vi "Database.Select.Variant.vi"(8 "error in":errorcluster, 9 "System":string="ST10", 10 "Variant":u64, 11 "Data in":T1 {"Variant"."TS"."TV"."minimum" format="%#.3f"; "Variant"."TS"."TV"."maximum" format="%#.3f"; "Variant"."TS"."TP"."value" format="%#.3f"}) -> (0 "error out":errorcluster, 3 "Data out":T1 {"Variant"."TS"."TV"."minimum" format="%#.3f"; "Variant"."TS"."TV"."maximum" format="%#.3f"; "Variant"."TS"."TP"."value" format="%#.3f"})   [LabVIEW 2016]
doc: "Write test results (measurement values) to proda database\n\nWabco 2017 All right reserved\nAuthor: maciej.szupienko@wabco-auto.com"
uses:
  Database.Main.Data.ctl
  Database.Main.Data.Status.ctl
  Database.Main.Data.Sets.ctl
  Database.Main.Data.Results.ctl
  ProdaNG/Controls/ProdaNG.Identification.ctl
  ProdaNG/Controls/ProdaNG.ProcessResult.ctl
  ProdaNG/Controls/ProdaNG.ProcessStepResult.ctl
  ProdaNG/Controls/ProdaNG.TestStepResult.ctl
  ProdaNG/Controls/ProdaNG.TestValueResult.ctl
  Database.Main.Data.Variant.ctl
  ProdaNG/Controls/ProdaNG.ProcessStepParam.ctl
  ProdaNG/Controls/ProdaNG.TestStep.ctl
  ProdaNG/Controls/ProdaNG.TestStepParam.ctl
  ProdaNG/Controls/ProdaNG.TestValue.ctl
  tools/Translator/Translator.Message.ctl
  tools/EventLog/EventLog.EventSource.ctl
  tools/EventLog/EventLog.New(single).vi
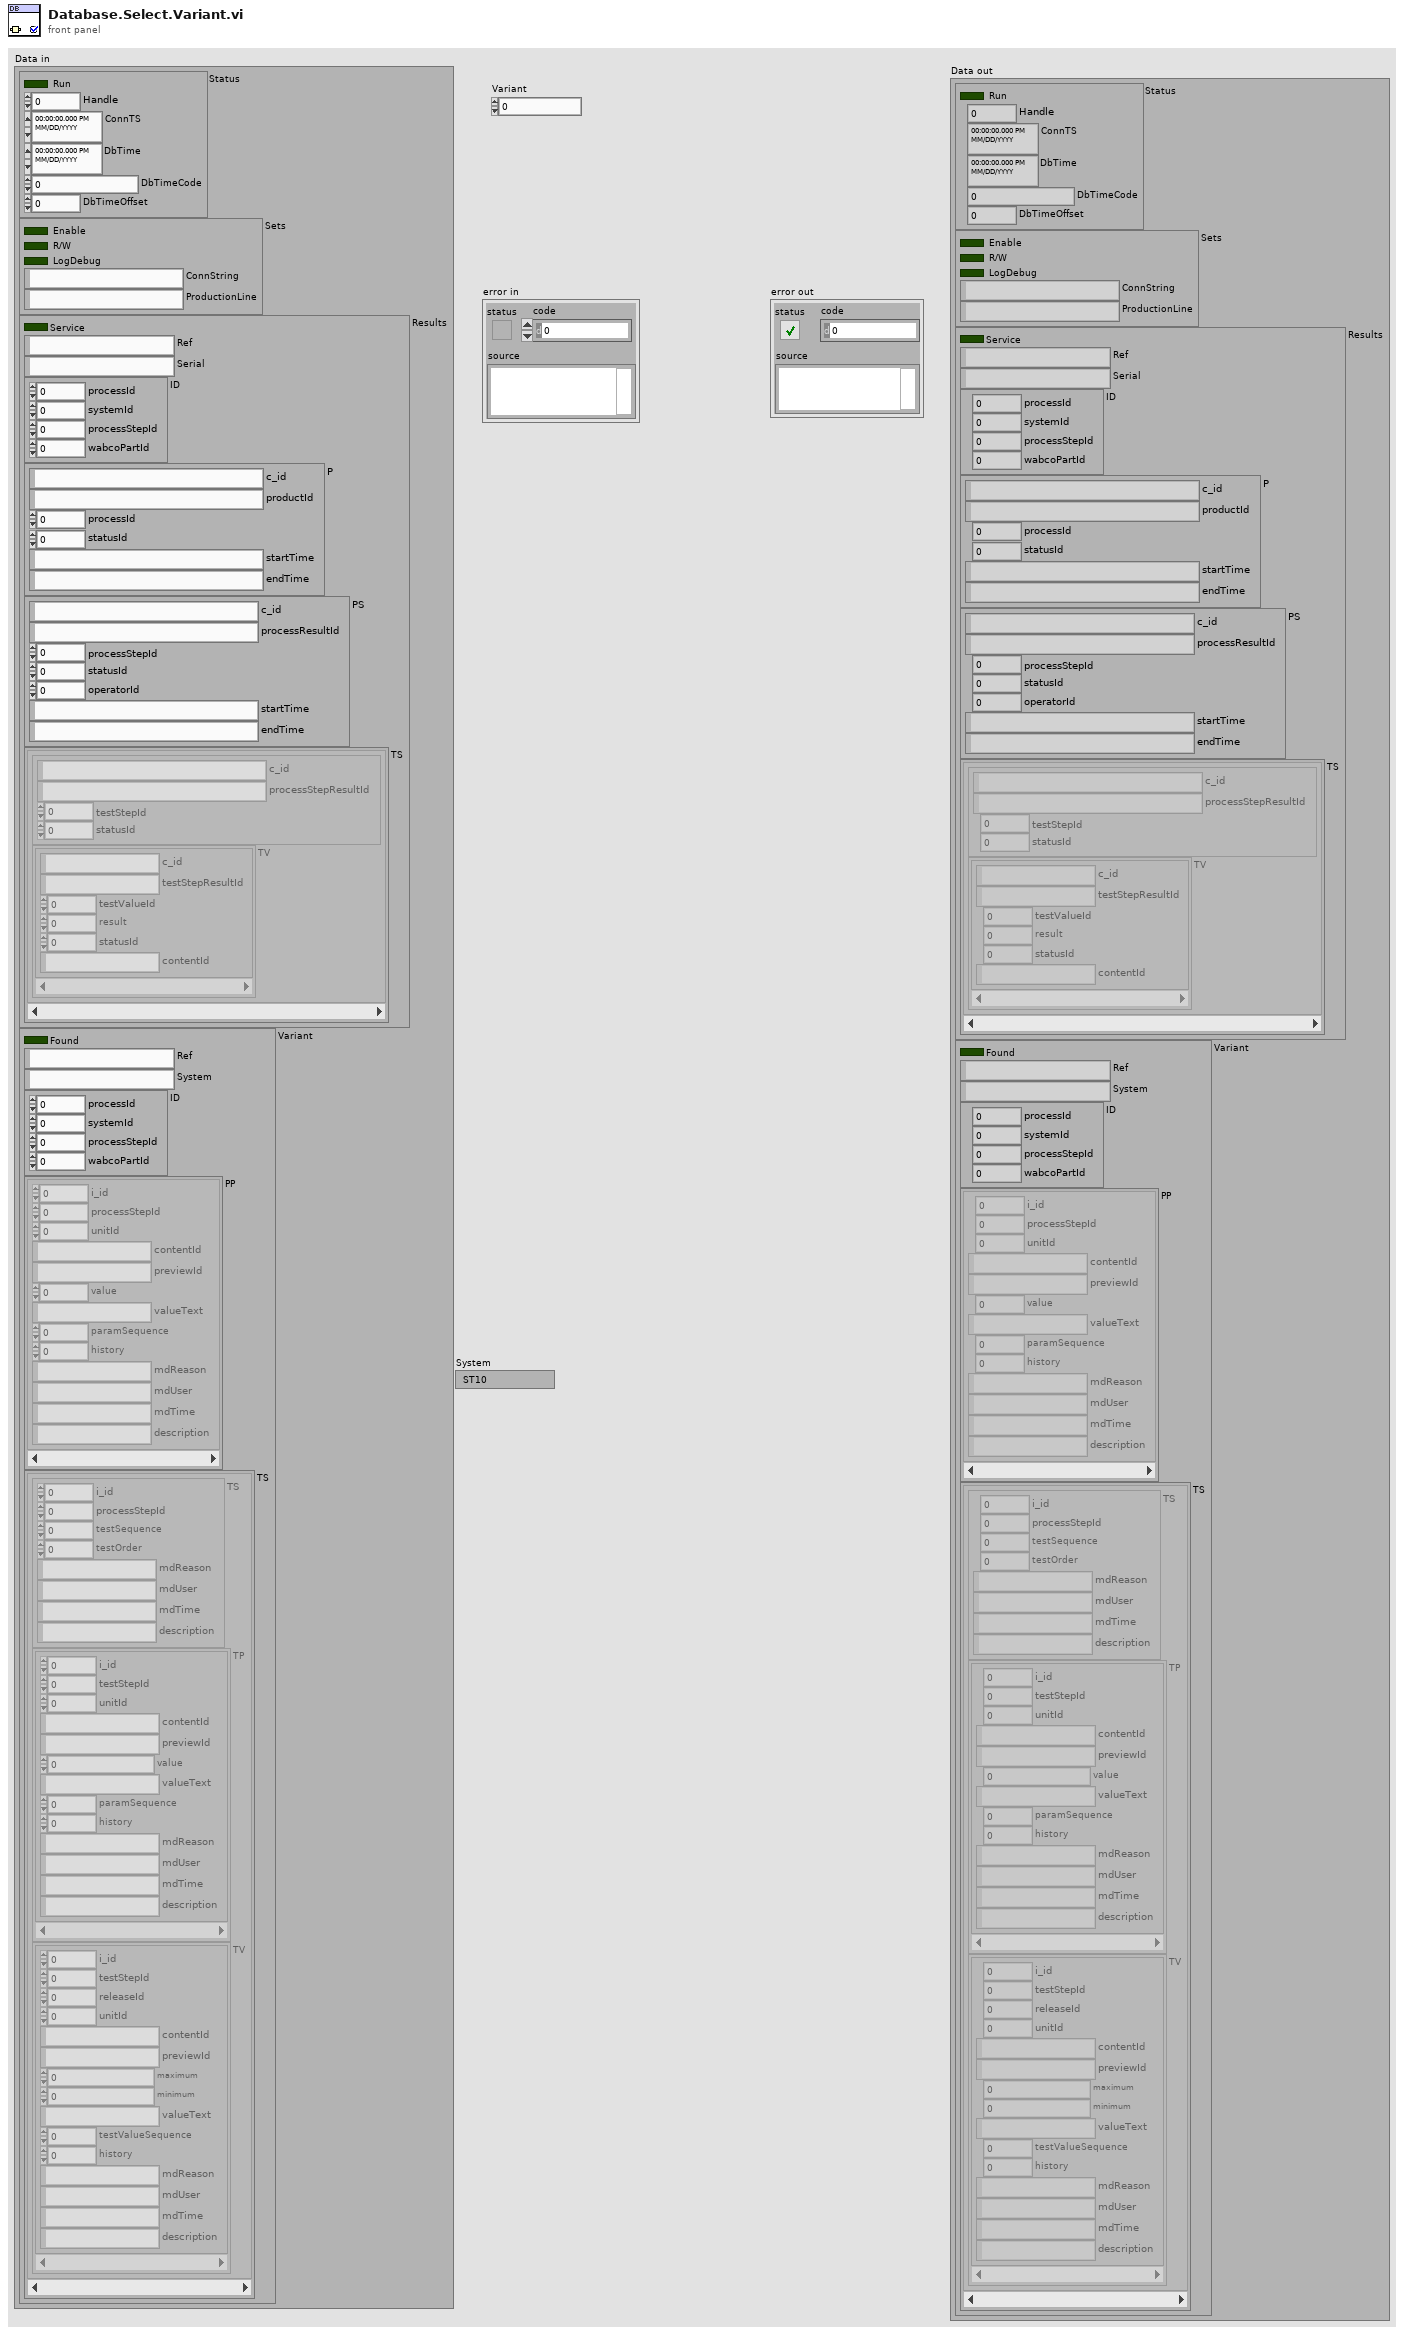
[diagram p1: front panel]
types:
  T1 = typedef "Database.Main.Data.ctl" = cluster{"Status":T2, "Sets":T3, "Results":T4, "Variant":T10}
  T2 = typedef "Database.Main.Data.Status.ctl" = cluster{"Run":bool, "Handle":i32, "ConnTS":timestamp, "DbTime":timestamp, "DbTimeCode":dbl, "DbTimeOffset":dbl}
  T3 = typedef "Database.Main.Data.Sets.ctl" = cluster{"Enable":bool, "R/W":bool, "LogDebug":bool, "ConnString":string, "ProductionLine":string}
  T4 = typedef "Database.Main.Data.Results.ctl" = cluster{"Service":bool, "Ref":string, "Serial":string, "ID":T5, "P":T6, "PS":T7, "TS":cluster{"TS":T8, "TV":T9[]}[]}
  T5 = typedef "ProdaNG.Identification.ctl" = cluster{"processId":i32, "systemId":i32, "processStepId":i32, "wabcoPartId":i32}
  T6 = typedef "ProdaNG.ProcessResult.ctl" = cluster{"c_id":string, "productId":string, "processId":i32, "statusId":i32, "startTime":string, "endTime":string}
  T7 = typedef "ProdaNG.ProcessStepResult.ctl" = cluster{"c_id":string, "processResultId":string, "processStepId":i32, "statusId":i32, "operatorId":i32, "startTime":string, "endTime":string}
  T8 = typedef "ProdaNG.TestStepResult.ctl" = cluster{"c_id":string, "processStepResultId":string, "testStepId":i32, "statusId":i32}
  T9 = typedef "ProdaNG.TestValueResult.ctl" = cluster{"c_id":string, "testStepResultId":string, "testValueId":i32, "result":dbl, "statusId":i32, "contentId":string}
  T10 = typedef "Database.Main.Data.Variant.ctl" = cluster{"Found":bool, "Ref":string, "System":string, "ID":T5, "PP":T11[], "TS":cluster{"TS":T12, "TP":T13[], "TV":T14[]}[]}
  T11 = typedef "ProdaNG.ProcessStepParam.ctl" = cluster{"i_id":i32, "processStepId":i32, "unitId":i32, "contentId":string, "previewId":string, "value":dbl, "valueText":string, "paramSequence":i32, "history":i32, "mdReason":string, "mdUser":string, "mdTime":string, "description":string}
  T12 = typedef "ProdaNG.TestStep.ctl" = cluster{"i_id":i32, "processStepId":i32, "testSequence":i32, "testOrder":i32, "mdReason":string, "mdUser":string, "mdTime":string, "description":string}
  T13 = typedef "ProdaNG.TestStepParam.ctl" = cluster{"i_id":i32, "testStepId":i32, "unitId":i32, "contentId":string, "previewId":string, "value":dbl, "valueText":string, "paramSequence":i32, "history":i32, "mdReason":string, "mdUser":string, "mdTime":string, "description":string}
  T14 = typedef "ProdaNG.TestValue.ctl" = cluster{"i_id":i32, "testStepId":i32, "releaseId":i32, "unitId":i32, "contentId":string, "previewId":string, "maximum":dbl, "minimum":dbl, "valueText":string, "testValueSequence":i32, "history":i32, "mdReason":string, "mdUser":string, "mdTime":string, "description":string}
  T15 = typedef "EventLog.EventSource.ctl" = enum16{"All", "Gui", "Ref", "File", "Arch", "Seq", "CPX", "DB", "Laser", "Scan.P", "Scan.O"}
  T16 = typedef "Translator.Message.ctl" = enum16{"-", "Event confirmed", "Log out", "Log in", "Shutdown", "Cancel", "Start", "Begin time", "End time", "Duration", "Service Mode", "Ignore Results", "Serial Format", "On", "Off", "OK", "NOK", "NOK %s", "Home", "Work", "Close", "Open", "In progress...", "Missing", "Empty", "Hardware failure", "Initial", "Default", "Total", "Out of range", "Free disk space is below 1GB - contact technician", "Error %d >> %s", "Error %d >> %s >> %s", "Msg %d >> %s", "Laser msg %d %s", "Laser cmd error %s %d", "Laser cmd failed %s", "Laser cmd warning %s", "Laser disconnected", "Laser status %s", "Laser already started", "Laser job unkonwn %s", "Laser job missing %s", "Laser job select failure %s", "Unable to start laser printing (%s)", "Unable to stop laser printing (%s)", "Laser marking aborted", "Laser marking timeout", "Unable to reset Laser Interlock (%s)", "Unable to trigger Laser. Laser not ready (%s)", "Laser job '%s' coordinates not configured", "Starting %s", "Quitting %s", "Configured", "Initializing", "Quitting", "Loading", "Loaded %d results", "Loaded %d events", "Running", "Stopped", "Summary", "Laser", "Do you want to continue?", "Do you want to delete the configuration?", "The configuration is being used by an order. Unable to delete!", "Press confirm button", "Station is not based. Do you want to exit?", "Station requires changeover. Do you want to run the test?", "Test options are not set as default. Do you want to continue?", "Formatting of WabcoNo is disabled. Do you want to continue?", "Product not detected. Do you want to continue?", "Product scan failed. Do you want to continue?", "Calibration", "Log out?", "System", "All", "IDLE", "Translating...%s", "Not found", "Alarm %s", "Run", "Skip", "Abort", "Repeat", "Please wait...", "Database disconnected", "Database disconnected - changeover disabled!", "Login to database successful", "Login to database failed: %d; %s", "Unable to check the product status of reference %d - database disconnected", "Unable to set the product status of reference %d - database disconnected", "Variant file backup %s", "Read variant (%s)", "Result", "Station armed!", "Station requires changeover!", "Select reference number...", "EMERGENCY BUTTON - press Control button", "EMERGENCY DOOR - press Control button", "Resetting Emergency...", "Unable to reset safety circuit - Emergency Button pressed", "Unable to reset safety circuit - Emergency Side Door open", "Station not based", "Station based", "Station not empty", "Station basing...", "No order", "Press Start to begin new order", "Scanning new order", "Order NOK. Correct or scan again", "Order OK. Press Accept", "Order ready", "Revolver incorrect", "Fork incorrect", "Revolver missing", "Revolver empty", "Container missing", "Offline results", "Offline statistics", "Updating statistics %.1f %%", "DMC Configurator", "Door open", "Close the front door", "Press start button", "Done. Open the front door", "Running...", "Running...%.1f %%", "Pause %s", "Pause %s. NOK container missing", "Pause %s. OK container missing", "Pause %s. Revolver empty", "Pause %s. Revolver missing", "Pause %s. Revolver incorrect", "Pause %s. Fork missing", "Pause %s. Fork incorrect", "Pause %s. Too many failures", "Pause %s. Unloading failure", "Pause %s. One slot is not working", "Pause %s. Part order is done. Empty OK container", "Pause %s. Unable to move product to slot", "Pause %s. Unable to move back product pusher", "Pause %s. Unable to lift product", "Pause %s. Unable to move back product lifter", "Pause %s. Unable to move product arm to Work", "Pause %s. Unable to move product arm to NOK", "Pause %s. Unable to move product arm to OK", "Pause %s. Unable to unsuck the NOK product", "Pause %s. Unable to drop the NOK product", "Pause %s. Product OK missing", "Pause %s. Unable to unsuck the OK product", "Pause %s. Unable to drop the OK product", "Stopping...", "File '%s' is missing", "File '%s' is broken", "File '%s' is running", "Log file started (%s)", "Log file ended (%s)", "Log file stopped (%s)", "Log file ignored (%s)", "Log file exported (%s)", "Log file export failed (%s)", "Wrong serial number in log file", "Wrong reference number in log file", "Test steps are missing", "%s = %.3f", "Process param '%s' not found in DB", "Process param '%s' wrong order", "Process param '%s' value %.3f out of limits (%.3f; %.3f)", "Step%d param '%s' not found in DB", "Step%d param '%s' wrong order", "Step%d param '%s' value %.3f out of limits (%.3f; %.3f)", "Step%d EV '%s' not found in DB", "Step%d EV '%s' wrong order", "\"%s\" not found in DB", "\"%s\" wrong order", "\"%s\" value %.3f out of limits (%.3f; %.3f)", "\"%s\" not found in software", "Process init (%s)", "Process started", "Process restarted", "Process run", "Process done", "Process done - remove OK container", "Process aborted", "Process aborted at work", "Process aborted at home", "Process error", "Process error at home", "Process error at work", "Process close", "Process pause", "Process continue", "Process door open", "Process door close", "Process pause at slot %s due to %s", "Select plate from the order to process", "Do you want to start the process?", "Do you want to continue the process?", "There is unfinished order. Do you want to put the new order?", "Product %s %d OK", "Product %s %d NOK", "Unable to unload the slot %s. Product missing in the slot", "Unable to unload the slot %s. Product already in the arm", "Unable to accept the product as OK. Product missing in slot %s", "Unable to accept the product as OK. Product could not drop into the container at slot %s", "Unable to accept the product as NOK. Product could not drop into the container at slot %s", "Scan failed. Error %s", "Scan failed. Scanner disconnected", "Scan failed. Wrong Wabco number %d, limit (%d,%d)", "Scan failed. Wrong serial number %d, limit (%d,%d)", "Scan failed. Wrong date %d, limit (%d,%d)", "Scan failed. Wrong product wabco number %d (expected %d)", "Scan failed. Wrong product serial number %d (expected > 0)", "Scan OK %s", "Scan failed. Unable to determine table position (%s)", "Scan failed. Timeout", "Tune failed. Scanner disconnected", "Tune failed. Timeout", "%s = %d", "%s = %d->%d", "Unable to set %s = %.2f - Air Pressure Inside off", "Unable to set digital output '%s' = %d", "Unable to activate air pressure inside - timeout", "Unable to activate air pressure inside - aborted", "Unable to switch on Air Main Valve - Air Pressure Inlet off", "Unable to switch on Air Main Valve - Door open", "Unable to switch off Air Main Valve - timeout", "Unable to switch off Air Main Valve - aborted", "Unable to rotate Table - timeout", "Unable to rotate Table - aborted", "Unable to rotate Table - Product Move not in Home position", "Unable to rotate Table - Air Pressure Inside off", "Unable to rotate Table - Product Lift A not in Home position", "Unable to rotate Table - Product Lift B not in Home position", "Unable to rotate Table - unlock before movement timeout", "Unable to rotate Table - lock after movement timeout", "Unable to move Table Lock to %s position - timeout", "Unable to move Table Lock to %s position - aborted", "Unable to move Table Lock to %s position - Air Pressure Inside off", "Unable to move Table Lock to %s position - Table not in position", "Unable to move Product Lift A to %s position - timeout", "Unable to move Product Lift B to %s position - timeout", "Unable to move Product Lift A to %s position - aborted", "Unable to move Product Lift B to %s position - aborted", "Unable to move Product Lift A to %s position - Air Pressure Inside off", "Unable to move Product Lift B to %s position - Air Pressure Inside off", "Unable to move Product Lift A to %s position - Table not locked", "Unable to move Product Lift B to %s position - Table not locked", "Unable to move Product Lift A to %s position - Product Arm not in Work position", "Unable to move Product Lift B to %s position - Product Arm not in Work position", "Unable to set Product Suction Gripper %s to %s - timeout", "Unable to set Product Suction Gripper %s to %s - aborted", "Unable to set Product Suction Gripper %s to %s - Air Pressure Inside off", "Unable to set Product Suction Gripper %s to %s - Table slot unkown", "Unable to move Product Arm to %s position - timeout", "Unable to move Product Arm to %s position - aborted", "Unable to move Product Arm to %s position - Air Pressure Inside off", "Unable to move Product Arm to %s position - Product Lift A not in Home position", "Unable to move Product Arm to %s position - Product Lift B not in Home position", "Unable to move Product to %s position - timeout", "Unable to move Product to %s position - aborted", "Unable to move Product to %s position - Air Pressure Inside off", "Unable to move Product to %s position - Table not in position"}
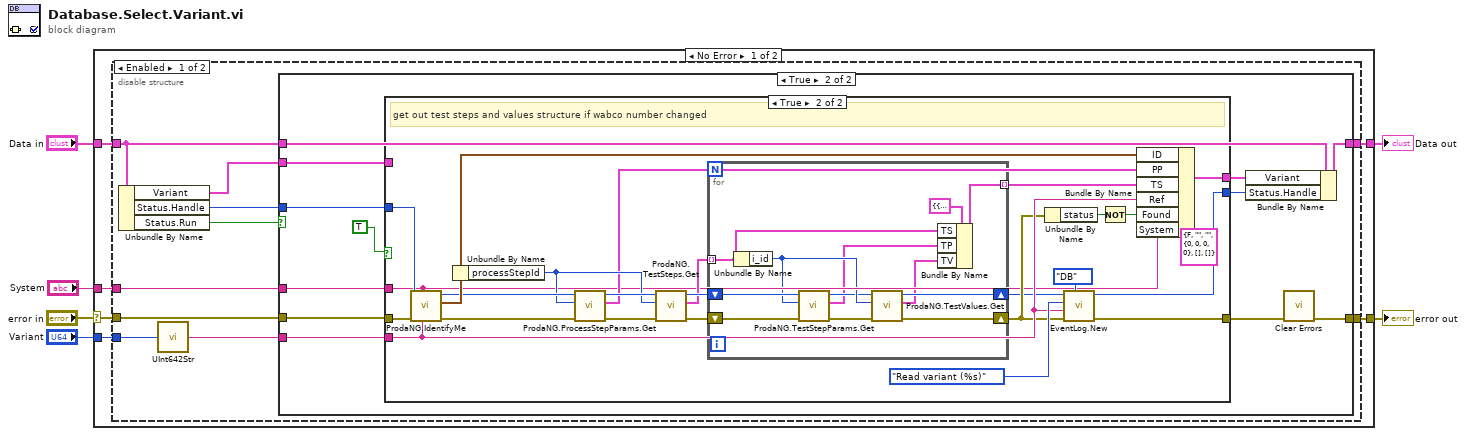
[diagram p0: block diagram]
diagram:
  n1 = case shown="No Error" "error in" {
    selector: "error in" -> [w12 w77]
    tunnel: [w9 w77] -> w6
    tunnel: "Data in" -> [w11 w76]
    tunnel: [w10 w76] -> w3
    tunnel: "Variant" -> [w8 _]
    tunnel: "System" -> [w7 _]
    frame No Error {
      n2 = disable-structure shown="Enabled" {
        disable-tunnel: w12 -> [w22 _]
        disable-tunnel: w11 -> [w20 _]
        disable-tunnel: [w19 _] -> w10
        disable-tunnel: [w17 _] -> w9
        disable-tunnel: w8 -> [w15 _]
        disable-tunnel: w7 -> [w13 _]
        frame Enabled {
          n3 = Unbundle By Name(w20) -> ("Variant"=w18:T10, "Status.Handle"=w21:i32, "Status.Run"=w14:bool)
          n4 = call "UInt642Str.vi"("Numeric"=w15) -> ("string"=w16:string)
          n5 = case shown="True" w14 {
            tunnel: w22 -> [w24 w36]
            tunnel: w13 -> [_ w25]
            tunnel: w21 -> [_ w35]
            tunnel: w16 -> [_ w28]
            tunnel: w20 -> [w23 w31]
            tunnel: [w23 w34] -> w19
            tunnel: w18 -> [_ w33]
            tunnel: [w24 w32] -> w17
            frame False {
            }
            frame True {
              n6 = case shown="True" TRUE {
                tunnel: w28 -> [_ w49]
                tunnel: w36 -> [w39 w60]
                tunnel: [w39 w58] -> w30
                tunnel: w35 -> [w38 w59]
                tunnel: [w38 w44] -> w27
                tunnel: w33 -> [w37 _]
                tunnel: [w37 w45] -> w29
                tunnel: w25 -> [_ w40]
                frame False {
                }
                frame True {
                  # "get out test steps and values structure if wabco number changed"
                  n7 = call "ProdaNG.IdentifyMe.vi"("wabcoNumber"=w49, "systemName"=w40, "error in"=w60, "dbHandleIn"=w59) -> ("error out"=w54:errorcluster, "Identification"=w62:T5, "dbHandle"=w55:i32)  [unwired: 5 in]
                  n8 = Unbundle By Name(w62) -> ("processStepId"=w51:i32)
                  n9 = call "ProdaNG.ProcessStepParams.Get.vi"("error in (no error)"=w54, "processStepId"=w51, "dbHandleIn"=w55) -> ("error out"=w52:errorcluster, "ProcStepParams"=w43:T11[], "dbHandle"=w53:i32)  [unwired: 6 in]
                  n10 = call "ProdaNG.TestSteps.Get.vi"("error in (no error)"=w52, "processStepId"=w51, "dbHandleIn"=w53) -> ("error out"=w61:errorcluster, "TestSteps"=w42:T12[], "dbHandle"=w63:i32)  [unwired: 6 in]
                  n11 = for {
                    tunnel: w42 -> [w72] mode=indexing
                    shift-right: [w75] -> w44
                    shift-left: w63 -> [w70]
                    shift-right: [w74] -> w48
                    shift-left: w61 -> [w66]
                    tunnel: [w64] -> w41 mode=indexing
                    n12 = Unbundle By Name(w72) -> ("i_id"=w69:i32)
                    n13 = call "ProdaNG.TestStepParams.Get.vi"("error in (no error)"=w66, "testStepId"=w69, "dbHandleIn"=w70) -> ("error out"=w68:errorcluster, "TestStepParams"=w65:T13[], "dbHandle"=w67:i32)  [unwired: 6 in]
                    n14 = call "ProdaNG.TestValues.Get.vi"("error in (no error)"=w68, "testStepId"=w69, "dbHandleIn"=w67) -> ("error out"=w74:errorcluster, "TestStepValues"=w71:T14[], "dbHandle"=w75:i32)  [unwired: 6 in]
                    n15 = Bundle By Name(cluster=cluster{"TS":T12, "TP":T13[], "TV":T14[]} {"TS"={"i_id"=0, "processStepId"=0, "testSequence"=0, "testOrder"=0, "mdReason"="", "mdUser"="", "mdTime"="", "description"=""}, "TP"=[], "TV"=[]} ("TS"), "TS"=w72, "TP"=w65, "TV"=w71) -> (w64:cluster{"TS":T12, "TP":T13[], "TV":T14[]})
                  }
                  n16 = Unbundle By Name(w48) -> ("status"=w47:bool)
                  n17 = call-poly "EventLog.New.vi"("Source (All)"=EventLog.EventSource."DB", "error in (no error)"=w48, "Arg"=w49, "Message (-)"=Translator.Message."Read variant (%s)") -> ("error out"=w58:errorcluster)  [unwired: 6 in, 1 out]
                  n18 = Not(x=w47) -> (.not. x?=w46:bool)
                  n19 = Bundle By Name(cluster=T10 {"Found"=FALSE, "Ref"="", "System"="", "ID"={"processId"=0, "systemId"=0, "processStepId"=0, "wabcoPartId"=0}, "PP"=[], "TS"=[]} ("Variant"), "ID"=w62, "PP"=w43, "TS"=w41, "Ref"=w49, "Found"=w46, "System"=w40) -> (w45:T10)
                }
              }
              n20 = Bundle By Name(cluster=w31, "Variant"=w29, "Status.Handle"=w27) -> (w34:T1)
              n21 = call <vilib>:"Clear Errors.vi"("error in (no error)"=w30) -> ("error out"=w32:errorcluster)  [unwired: 5 in, 1 out]
            }
          }
        }
        frame Disabled {
        }
      }
    }
    frame Error {
    }
  }
  "error out" <- w6
  "Data out" <- w3
